vi "Settings Editor.vi"(8 "Error In":errorcluster) -> (0 "Error Out":errorcluster)   [LabVIEW 2022 SP3]
doc: "This VI is the Settings Editor or the \"New VI From Template\" tool.\n\nIt enables the user to view and change settings stored in the Windows Registry.\n\nAlternatively, the user can of course use the Windows Registry Editor to change the settings."
panel:
  out "Loop Iteration":i32
  in  "Save Button":bool
  in  "\"Open FP When Created?\" ticked by default?":enum32{"Yes", "No"}(radio) caption="\"Open Front Panel When Created?\" ticked by default?"
  in  "Templates Folder Location":path
  # "The template VI's and CTL's are expected to be found inside this folder."
  # "The settings are stored in the Windows Registry:\nHKEY_CURRENT_USER\\Software\\NewViFromTemplate_LabVIEW_IDE_Extension"
  # "The section below is for developer use only."
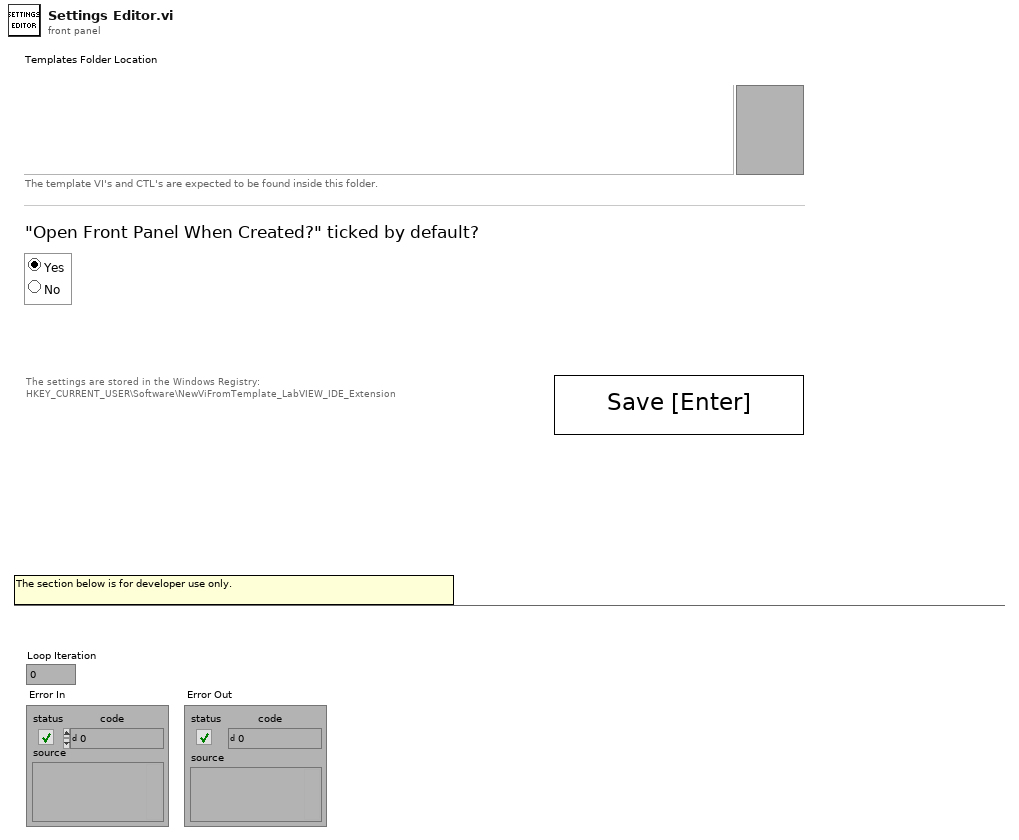
[diagram p1: front panel]
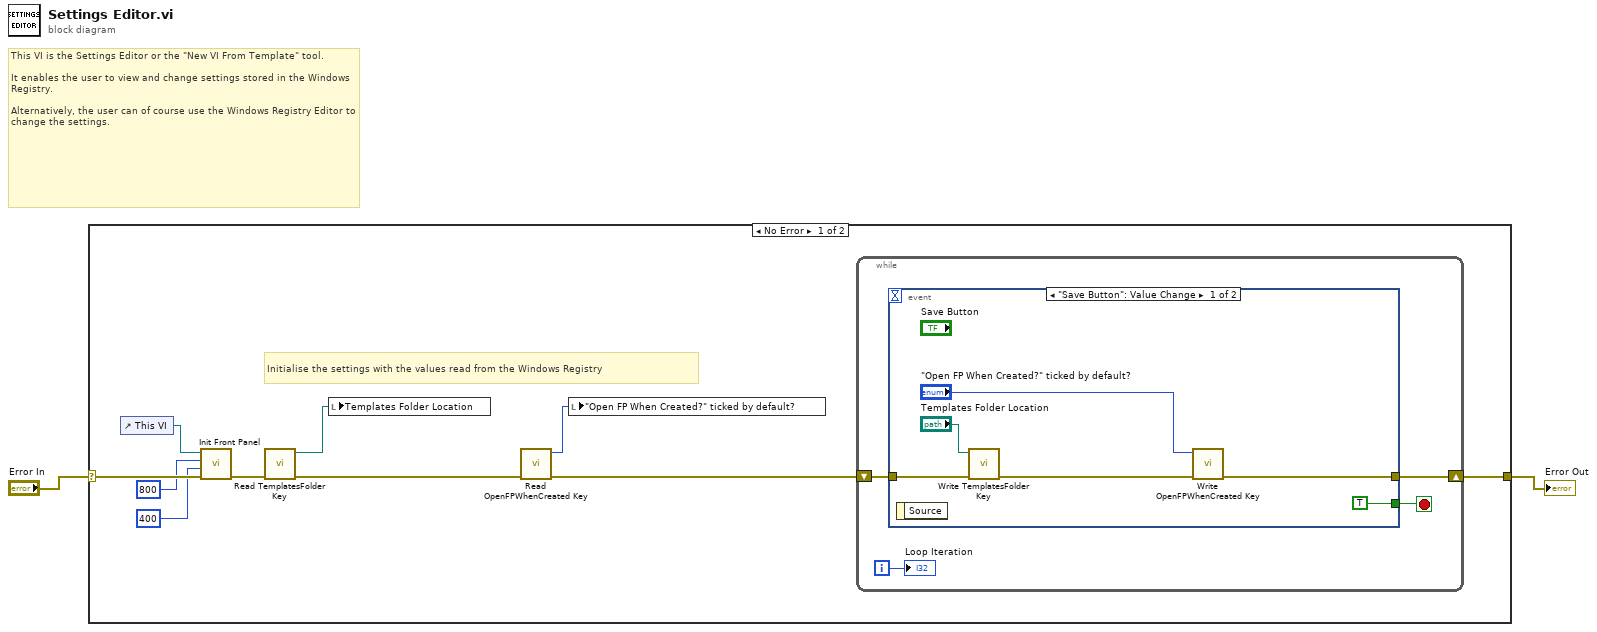
[diagram p0: block diagram]
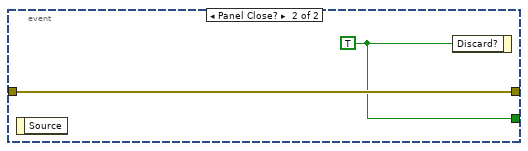
[diagram p2: hidden frame]
diagram:
  # "This VI is the Settings Editor or the \"New VI From Template\" tool.\n\nIt enables the user to view and change settings stored in the Windows Registry.\n\nAlternatively, the user can of course use the Windows Registry Editor to change the settings."
  n1 = case shown="No Error" "Error In" {
    selector: "Error In" -> [w12 w25]
    tunnel: [w8 w25] -> w1
    frame No Error {
      # "Initialise the settings with the values read from the Windows Registry"
      n2 = control-ref of="This VI"() -> (w11:refnum<vi>)
      n3 = call "Init Front Panel.vi"("error in"=w12, "Vertical Size (pixels)"=i16 400, "Horizontal Size (pixels)"=i16 800, "VI Reference"=w11) -> ("error out"=w7:errorcluster)  [unwired: 7 in]
      n4 = call "Read TemplatesFolder Key.vi"("Error In"=w7) -> ("Error Out"=w5:errorcluster, "Templates Folder Path"=w6:path)  [unwired: 9 in]
      n5 = local write "Templates Folder Location"(w6) -> ()
      n6 = call "Read OpenFPWhenCreated Key.vi"("Error In"=w5) -> ("Error Out"=w4:errorcluster, "Open Front Panel When Created?"=w3:enum32{"Yes", "No"})  [unwired: 9 in]
      n7 = local write "\"Open FP When Created?\" ticked by default?"(w3) -> ()
      n8 = while {
        shift-right: [w15] -> w8
        shift-left: w4 -> [w16]
        i -> [w13]
        stop <- w14 stop-if-true
        n9 = event shown="[0] \"Save Button\": Value Change" {
          selector: _ -> [_ _]
          dyn-events: _ -> [_ _]
          timeout: _ -> [_ _]
          tunnel: w16 -> [w21 w24]
          tunnel: [w18 w24] -> w15
          tunnel: [TRUE w23] -> w14
          event "Save Button": Value Change {
            n10 = event-data() -> ()  [unwired: 1 in, 1 out]
            n11 = call "Write TemplatesFolder Key.vi"("Error In"=w21, "Templates Folder Path"="Templates Folder Location") -> ("Error Out"=w19:errorcluster)  [unwired: 9 in]
            n12 = call "Write OpenFPWhenCreated Key.vi"("Error In"=w19, "\"Open FP When Created?\" ticked by default?"="\"Open FP When Created?\" ticked by default?") -> ("Error Out"=w18:errorcluster)  [unwired: 9 in]
          }
          event Panel Close? {
            w23 = TRUE ("Discard?")
            n13 = event-data() -> ()  [unwired: 1 in, 1 out]
            n14 = event-data("Discard?"=w23) -> ()  [unwired: 1 in, 1 out]
          }
        }
        "Loop Iteration" <- w13
      }
    }
    frame Error {
    }
  }
  "Error Out" <- w1
